vi "Configuration - DMM Properties FGV.vi"(8 "error in (no error)":errorcluster, 11 "Configuration Group of Channels Ref In":T1 format="%.0x") -> (0 "error out":errorcluster, 3 "Configuration Group of Channels Ref Out":T1 format="%.0x")   [LabVIEW 2016, in "DMM-SWITCH-ScanList System Explorer.lvlib"]
uses:
  DMM-SWITCH-ScanList System Explorer.lvlib
  <vilib>/NI Veristand/Custom Device API/Custom Device Item Ref.ctl
  <vilib>/NI Veristand/Custom Device API/Custom Device Channel.ctl
  <vilib>/NI Veristand/Custom Device API/Custom Device Channel Type.ctl
  Shared/Constants.vi
  <vilib>/NI Veristand/Custom Device API/Set Item Property (String).vi
  <vilib>/NI Veristand/Custom Device API/Set Item Property (U16).vi
  <vilib>/NI Veristand/Custom Device API/Set Item Property (Double).vi
  <vilib>/NI Veristand/Custom Device API/Set Item Property (Variant).vi
  <vilib>/NI Veristand/Custom Device API/Custom Device API.lvlib
  Shared/DMM-SWITCH-ScanList Shared.lvlib
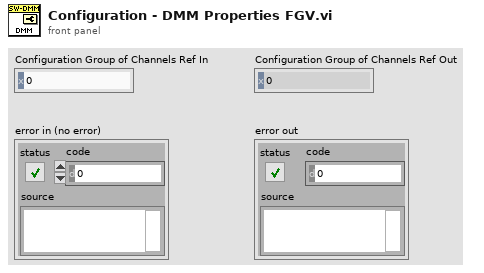
[diagram p1: front panel]
types:
  T1 = typedef "Custom Device API.lvlib/Custom Device Item Ref.ctl" = u64
  T2 = typedef "Custom Device API.lvlib/Custom Device Channel.ctl" = cluster{"Type":T3, "Units":string, "Default Value":dbl, "Faultable":bool, "Scalable":bool}
  T3 = typedef "Custom Device API.lvlib/Custom Device Channel Type.ctl" = enum16{"Input", "Output"}
  T4 = typedef "niDMM Function.ctl" = enum16{"DC Volts", "AC Volts", "DC Current", "AC Current", "2-wire Resistance", "4-wire Resistance", "Diode", "Frequency", "Period", "AC Volts DC Coupled", "Capacitance", "Inductance", "Temperature"}
  T5 = typedef "niDMM Resolution in Digits.ctl" = dbl
  T6 = typedef "DMM-SWITCH-ScanList System Explorer.lvlib/DMM Temp.ctl" = cluster{"DMM Temp - Transducer Type":T7, "DMM Temp - Thermocouple Type":T8, "DMM Temp - Fixed Reference Junction":dbl, "DMM Temp - RTD Type":T9, "DMM Temp - RTD Resistance":dbl, "DMM Temp - Thermistor Type":T10, "DMM Temp - RTD A":dbl, "DMM Temp - RTD B":dbl, "DMM Temp - RTD C":dbl, "DMM Temp - Thermistor A":dbl, "DMM Temp - Thermistor B":dbl, "DMM Temp - Thermistor C":dbl}
  T7 = typedef "niDMM Transducer Type.ctl" = i32
  T8 = typedef "niDMM Thermocouple Type.ctl" = i32
  T9 = typedef "niDMM RTD Type.ctl" = enum16{"Custom", "Pt3750", "Pt3851", "Pt3911", "Pt3916", "Pt3920", "Pt3928"}
  T10 = typedef "niDMM Thermistor Type.ctl" = enum16{"Custom", "44004", "44006", "44007"}
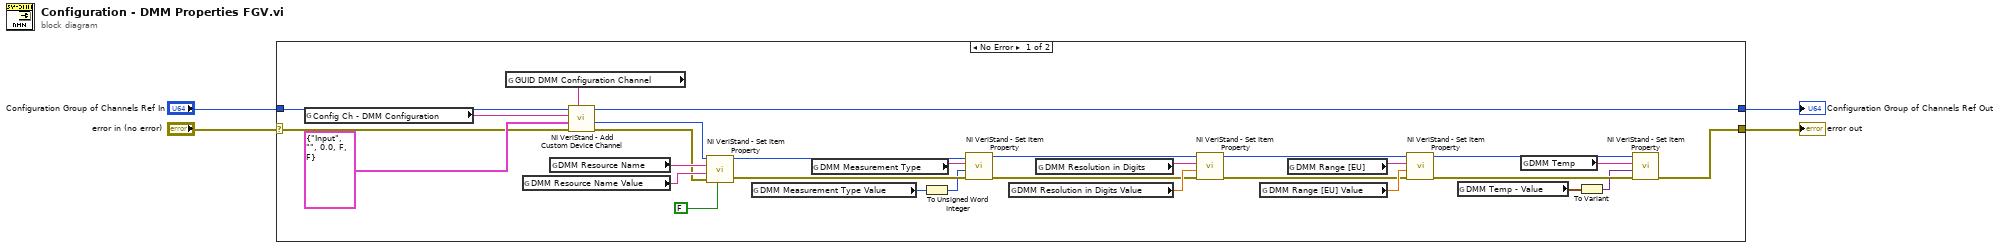
[diagram p0: block diagram]
diagram:
  n1 = case shown="No Error" "error in (no error)" {
    selector: "error in (no error)" -> [w12 w35]
    tunnel: [w7 w35] -> w4
    tunnel: [w14 w36] -> w3
    tunnel: "Configuration Group of Channels Ref In" -> [w13 w36]
    frame No Error {
      n2 = global read "Constants.vi" "Config Ch - DMM Configuration"() -> (w11:string)
      n3 = global read "Constants.vi" "GUID DMM Configuration Channel"() -> (w30:string)
      n4 = global read "Constants.vi" "DMM Resource Name Value"() -> (w26:string)
      n5 = global read "Constants.vi" "DMM Resource Name"() -> (w31:string)
      n6 = call <vilib>:"NI VeriStand - Add Custom Device Channel.vi"("GUID (Default Channel)"=w30, "error in (no error)"=w12, "Channel"=T2 {"Type"=enum."Input", "Units"="", "Default Value"=0.0, "Faultable"=FALSE, "Scalable"=FALSE}, "Channel Name"=w11, "Parent Ref in"=w13) -> ("error out"=w23:errorcluster, "Channel Ref"=w15:T1, "Parent Ref out"=w14:T1)  [unwired: 3 in, 1 out]
      n7 = call-poly <vilib>:"NI VeriStand - Set Item Property.vi"("Binary String (T)"=FALSE, "error in (no error)"=w23, "Value"=w26, "Property Name"=w31, "Item Ref in"=w15) -> ("error out"=w17:errorcluster, "Item Ref out"=w18:T1)  [unwired: 4 in, 1 out]
      n8 = global read "Constants.vi" "DMM Measurement Type Value"() -> (w27:T4)
      n9 = global read "Constants.vi" "DMM Measurement Type"() -> (w32:string)
      n10 = To Unsigned Word Integer(number=w27) -> (unsigned 16bit integer=w16:u16)
      n11 = call-poly <vilib>:"NI VeriStand - Set Item Property.vi"("error in (no error)"=w17, "Value"=w16, "Property Name"=w32, "Item Ref in"=w18) -> ("error out"=w20:errorcluster, "Item Ref out"=w19:T1)  [unwired: 5 in, 1 out]
      n12 = global read "Constants.vi" "DMM Resolution in Digits Value"() -> (w28:T5)
      n13 = global read "Constants.vi" "DMM Resolution in Digits"() -> (w33:string)
      n14 = call-poly <vilib>:"NI VeriStand - Set Item Property.vi"("error in (no error)"=w20, "Value"=w28, "Property Name"=w33, "Item Ref in"=w19) -> ("error out"=w22:errorcluster, "Item Ref out"=w21:T1)  [unwired: 5 in, 1 out]
      n15 = global read "Constants.vi" "DMM Range [EU] Value"() -> (w29:dbl)
      n16 = global read "Constants.vi" "DMM Range [EU]"() -> (w34:string)
      n17 = call-poly <vilib>:"NI VeriStand - Set Item Property.vi"("error in (no error)"=w22, "Value"=w29, "Property Name"=w34, "Item Ref in"=w21) -> ("error out"=w8:errorcluster, "Item Ref out"=w9:T1)  [unwired: 5 in, 1 out]
      n18 = global read "Constants.vi" "DMM Temp - Value"() -> (w6:T6)
      n19 = global read "Constants.vi" "DMM Temp"() -> (w10:string)
      n20 = To Variant(anything=w6) -> (Variant=w5:variant)
      n21 = call-poly <vilib>:"NI VeriStand - Set Item Property.vi"("error in (no error)"=w8, "Value"=w5, "Property Name"=w10, "Item Ref in"=w9) -> ("error out"=w7:errorcluster)  [unwired: 5 in, 2 out]
    }
    frame Error {
    }
  }
  "error out" <- w4
  "Configuration Group of Channels Ref Out" <- w3
